vi "Spectrograph_acceptCommand_changeDisperser.vi"(8 "error in (no error)":errorcluster, 11 "command_changeDisperser_Ctl":T1) -> (0 "error out":errorcluster, 2 "function return":i32, 3 "command_changeDisperser_Ctl out":T1)   [LabVIEW 2016, in "SALLV_Spectrograph.lvlib"]
doc: "int Spectrograph_shm_acceptCommand_changeDisperserLV(Spectrograph_command_changeDisperserLV *command_changeDisperser_Ctl );"
uses:
  SALLV_Spectrograph.lvlib
  DataTypes/command_changeDisperser.ctl
  SALLV_Spectrograph.so
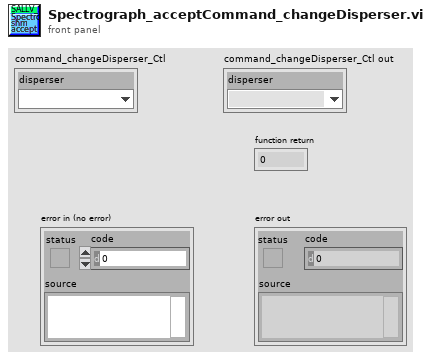
[diagram p1: front panel]
types:
  T1 = typedef "SALLV_Spectrograph.lvlib/command_changeDisperser.ctl" = cluster{"disperser":enum32{"", "disperser0", "disperser1", "disperser2", "disperser3"}}
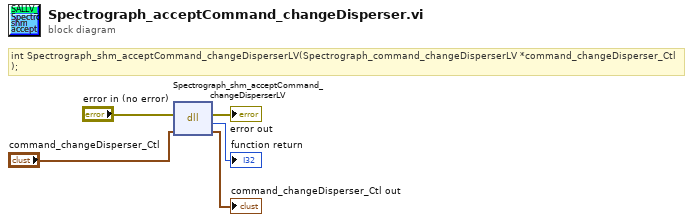
[diagram p0: block diagram]
diagram:
  # "int Spectrograph_shm_acceptCommand_changeDisperserLV(Spectrograph_command_changeDisperserLV *command_changeDisperser_Ctl );"
  n1 = dll-call lib="home/harini/TCS/SALLV_Spectrograph/SALLV_Spectrograph.*" fn="Spectrograph_shm_acceptCommand_changeDisperserLV"(error in="error in (no error)", "command_changeDisperser_Ctl"="command_changeDisperser_Ctl") -> (error out=→"error out":errorcluster, →"function return":i32, "command_changeDisperser_Ctl"=→"command_changeDisperser_Ctl out":T1)  [unwired: 2 in, 1 out]
